vi "Remove Vi.vi"(8 "error in":errorcluster caption="错误输入（无错误）", 9 "Abort VI":bool, 11 "PanelDataNode 输入":refnum<class "PanelDataNode.lvclass"> caption="DNL_LabVIEW Object in") -> (0 "error out":errorcluster caption="错误输出", 1 "VI*":refnum<vi>, 2 "ViValue":string, 3 "PanelDataNode 输出":refnum<class "PanelDataNode.lvclass"> caption="DNL_LabVIEW Object out")   [LabVIEW 2013, in "PanelDataNode.lvclass"]
uses:
  PanelDataNode.lvclass
  PanelDataNode.lvclass/PanelDataNode.ctl
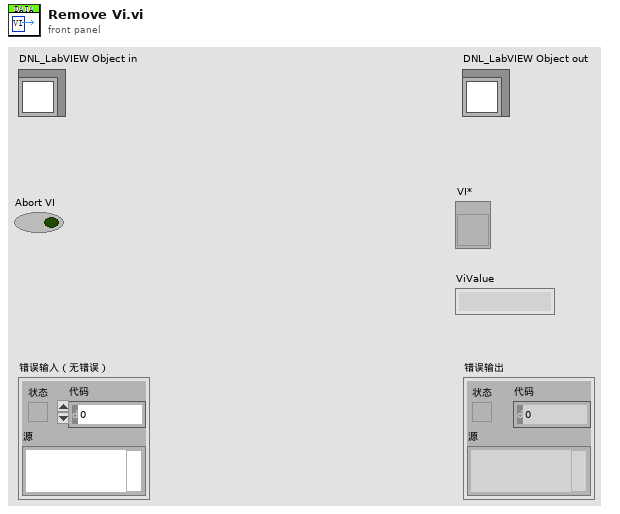
[diagram p1: front panel]
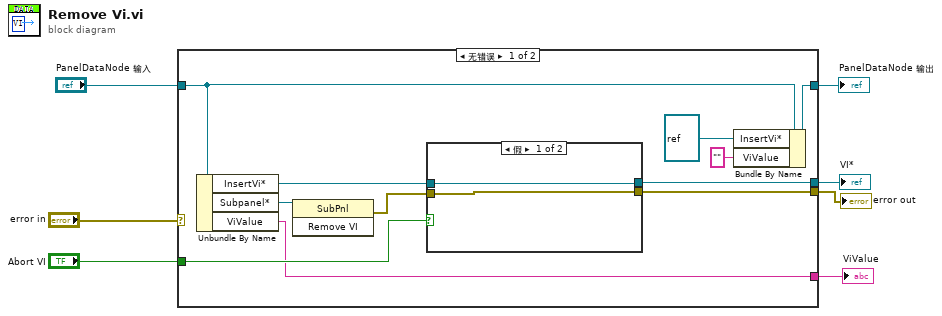
[diagram p0: block diagram]
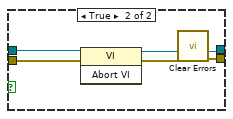
[diagram p2: hidden frame]
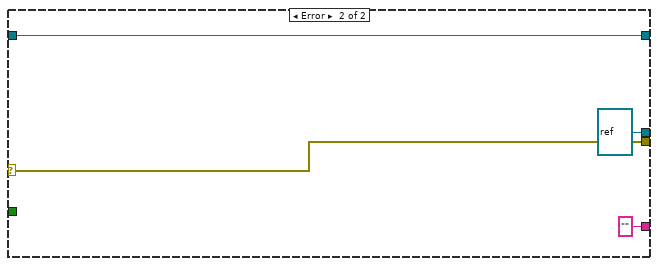
[diagram p3: hidden frame]
diagram:
  n1 = case shown="无错误" "error in" {
    selector: "error in" -> [_ w29]
    tunnel: [w10 w29] -> w6
    tunnel: [w13 w28] -> w4
    tunnel: "PanelDataNode 输入" -> [w14 w28]
    tunnel: [w15 refnum<vi> refnum ("VI*")] -> w3
    tunnel: "Abort VI" -> [w16 _]
    tunnel: [w8 "" ("ViValue")] -> w1
    frame No Error {
      n2 = Unbundle By Name(w14) -> ("InsertVi*"=w17:refnum<vi>, "Subpanel*"=w18:refnum<vi>, "ViValue"=w8:string)
      n3 = invoke class="SubPnl" method="Remove VI"(reference=w18) -> (error out=w11:errorcluster)  [unwired: 2 in, 2 out]
      n4 = case shown="假" w16 {
        tunnel: w17 -> [w20 w22]
        tunnel: [w20 w25] -> w15
        tunnel: [w19 w23] -> w10
        tunnel: w11 -> [w19 w21]
        frame False {
        }
        frame True {
          n5 = invoke class="VI" method="Abort VI"(reference=w22, error in=w21) -> (reference out=w25:refnum<vi>, error out=w24:errorcluster)  [unwired: 1 in, 1 out]
          n6 = call <vilib>:"Clear Errors.vi"("error in (no error)"=w24) -> ("error out"=w23:errorcluster)  [unwired: 6 in]
        }
      }
      n7 = Bundle By Name(cluster=w14, "InsertVi*"=refnum<vi> refnum ("VI*"), "ViValue"="") -> (w13:refnum<class "PanelDataNode.lvclass">)
    }
    frame Error {
    }
  }
  "error out" <- w6
  "PanelDataNode 输出" <- w4
  "VI*" <- w3
  "ViValue" <- w1
